vi "OBD_init.vi"(8 "error in":errorcluster, 10 "COM port":refnum<visa-resource-name>="COM2", 11 "cluster input":T1) -> (0 "error out":errorcluster, 2 "OBD enabled":bool=TRUE, 3 "cluster output":T1)   [LabVIEW 2020]
doc: "Initialize OBD communication"
uses:
  controls/StateMachineVariables.ctl
  <vilib>/vision/Avi.llb/IMAQ AVI2 Refnum.ctl
  <vilib>/userDefined/High Color/IMAQdx.ctl
  <vilib>/vision/Deep Learning.llb/IMAQ DL Model Refnum.ctl
  <vilib>/vision/Image Controls.llb/IMAQ Image.ctl
  <vilib>/Instr/_visa.llb/VISA Configure Serial Port (Instr).vi
  terminal_test.vi
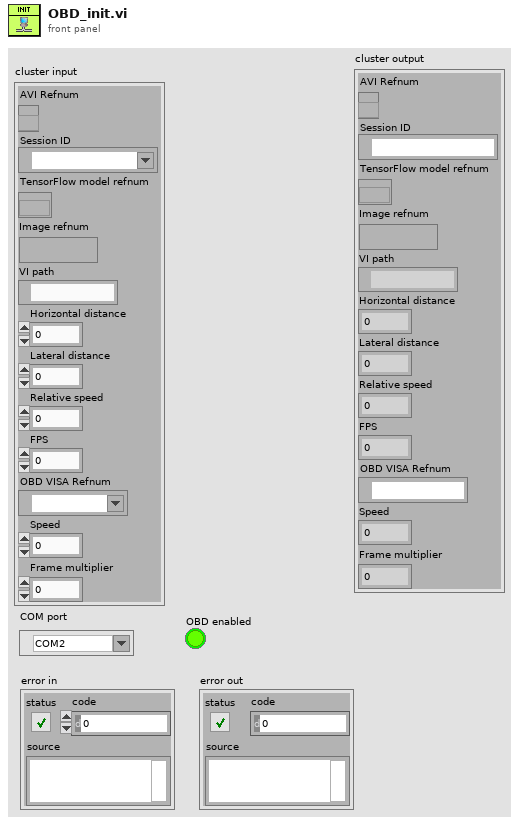
[diagram p1: front panel]
types:
  T1 = typedef "StateMachineVariables.ctl" = cluster{"AVI Refnum":T2, "Session ID":T3, "TensorFlow model refnum":T4, "Image refnum":T5, "VI path":path, "Horizontal distance":dbl, "Lateral distance":dbl, "Relative speed":dbl, "FPS":dbl, "OBD VISA Refnum":refnum<visa-resource-name>, "Speed":dbl, "Frame multiplier":u32}
  T2 = typedef "IMAQ AVI2 Refnum.ctl" = refnum<k20>
  T3 = typedef "IMAQdx.ctl" = refnum<k21>
  T4 = typedef "IMAQ DL Model Refnum.ctl" = refnum<k20>
  T5 = typedef "IMAQ Image.ctl" = refnum<image>
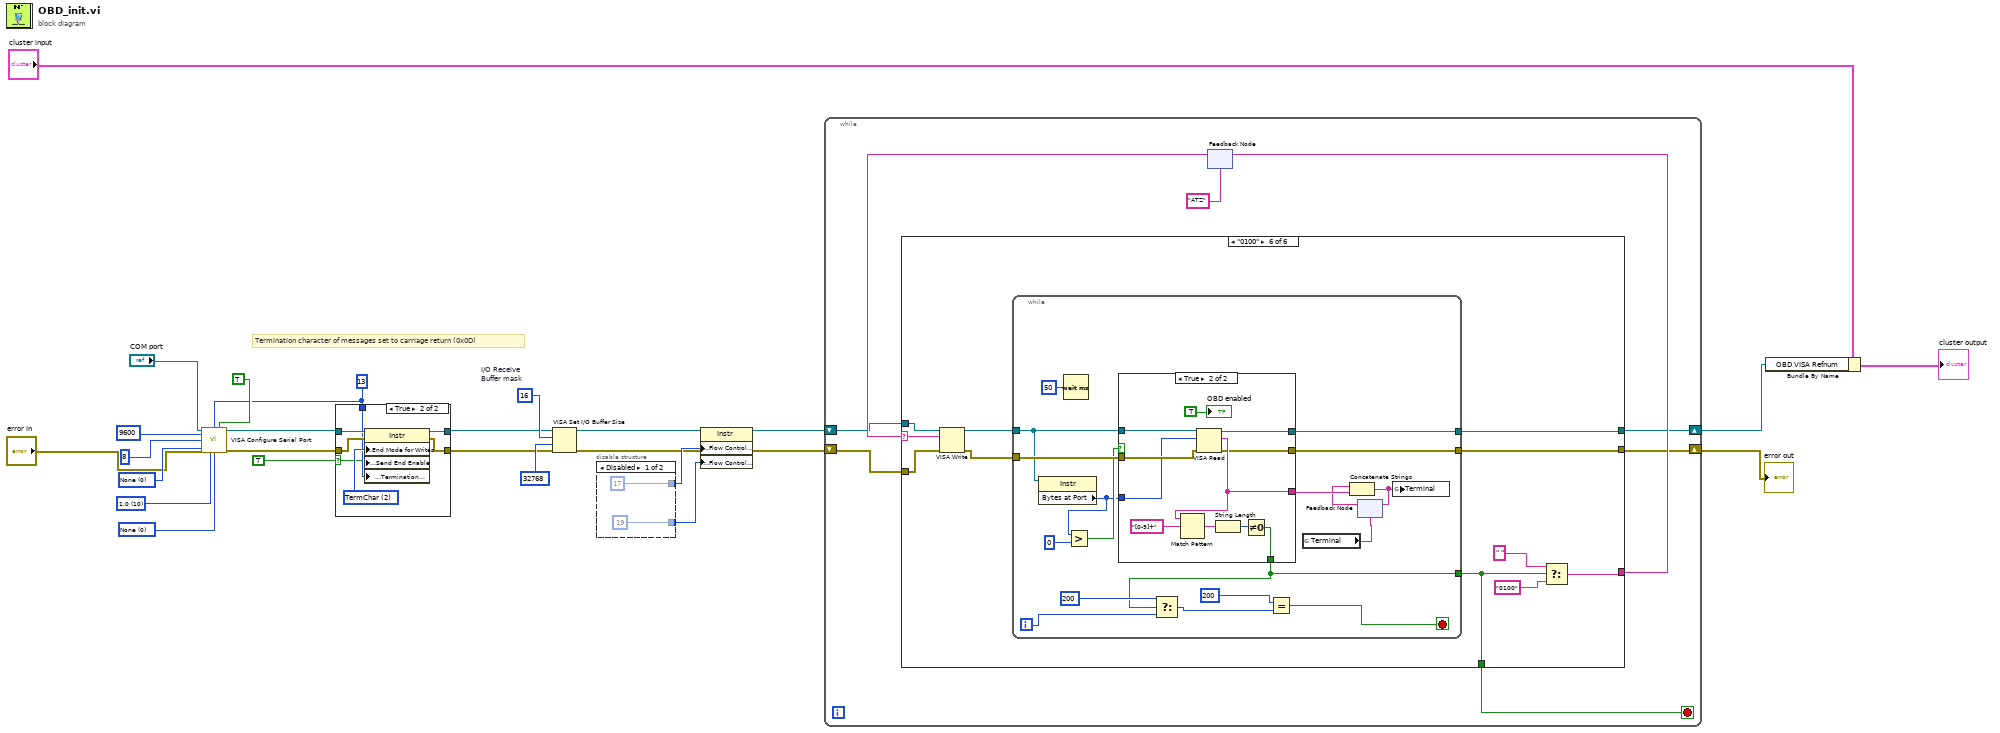
[diagram p0: block diagram]
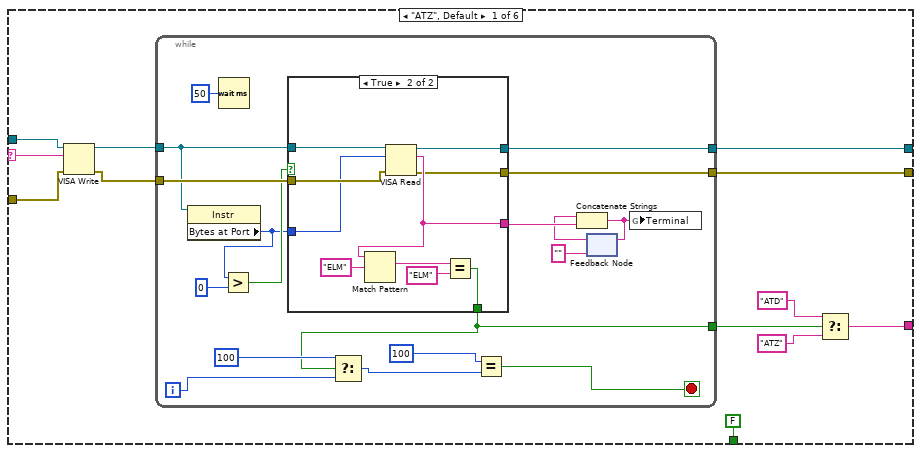
[diagram p4: hidden frame]
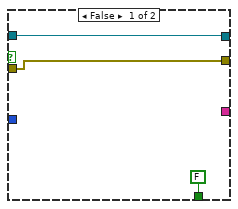
[diagram p5: hidden frame]
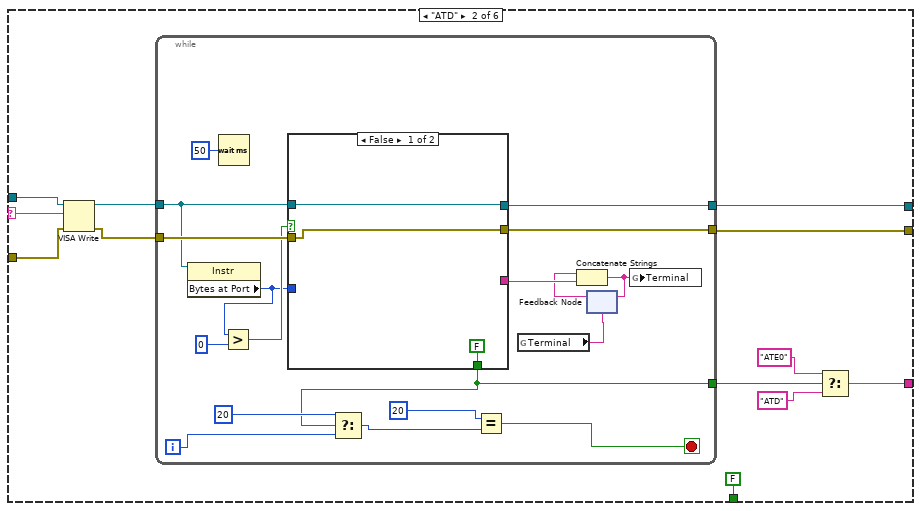
[diagram p6: hidden frame]
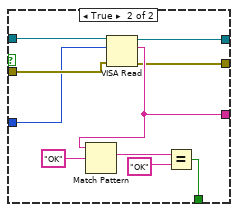
[diagram p7: hidden frame]
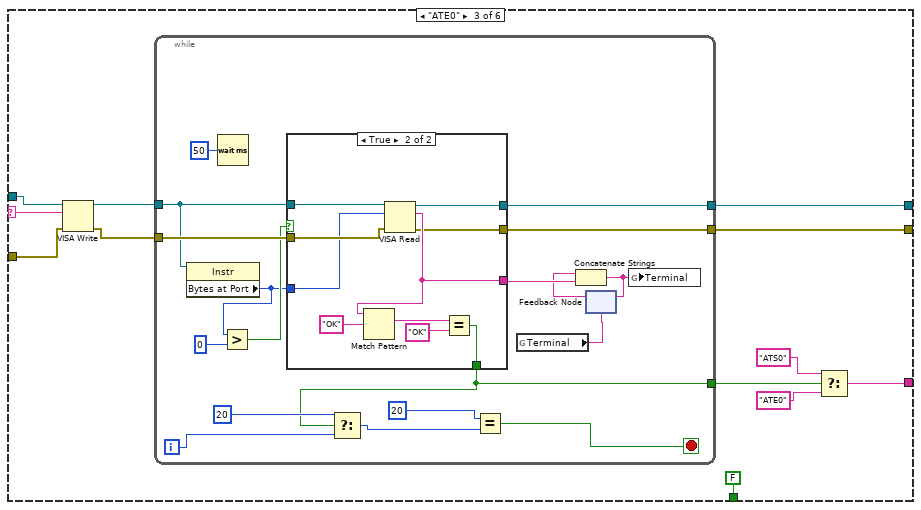
[diagram p8: hidden frame]
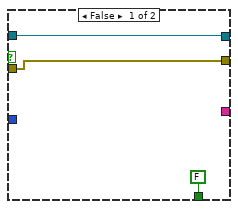
[diagram p9: hidden frame]
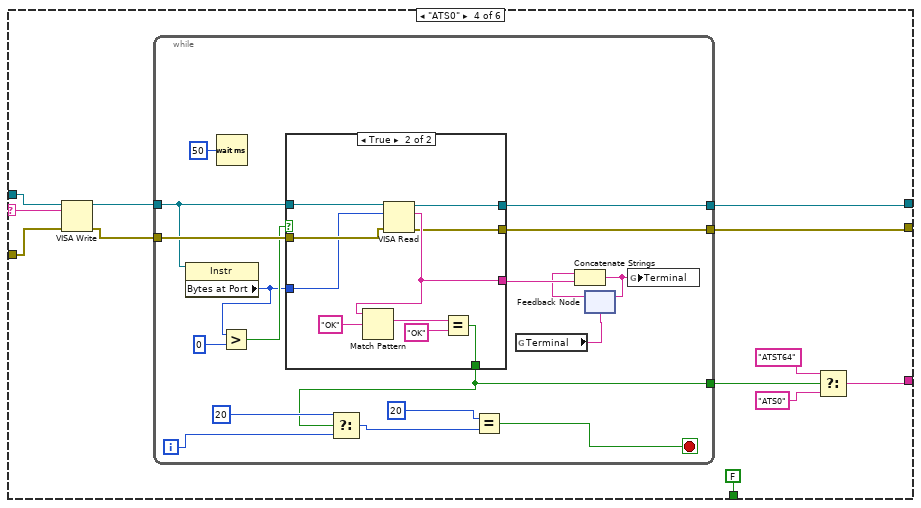
[diagram p10: hidden frame]
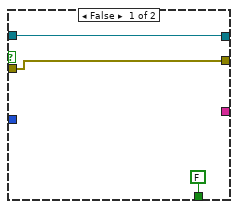
[diagram p11: hidden frame]
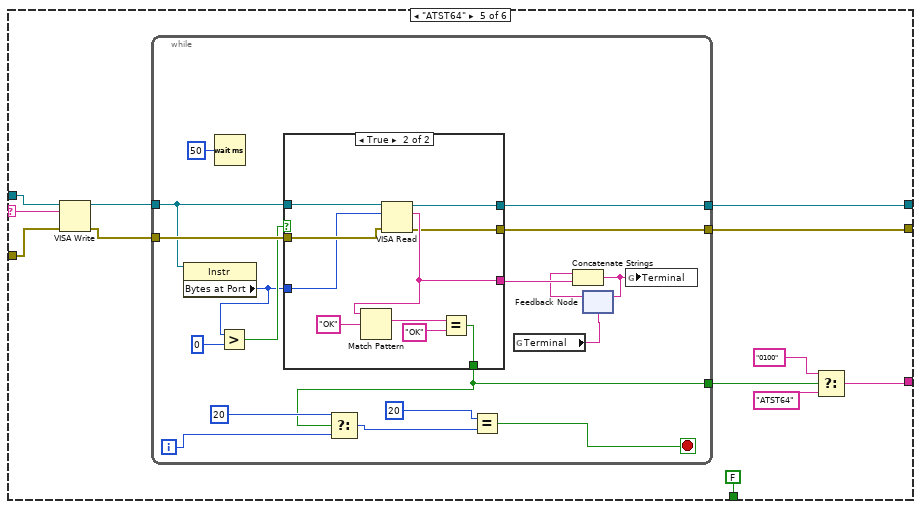
[diagram p12: hidden frame]
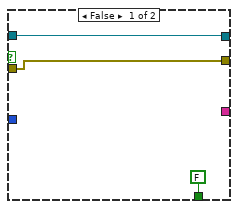
[diagram p13: hidden frame]
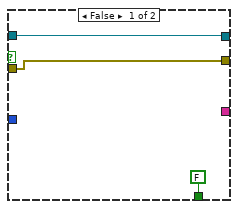
[diagram p14: hidden frame]
diagram:
  w18 = u16 0 items=["None"=0, "XON/XOFF"=1, "RTS/CTS"=2, "DTR/DSR"=4] ("flow control")
  w22 = u16 10 items=["1.0"=10, "1.5"=15, "2.0"=20] ("stop bits")
  w12 = u8 13 ("termination char\n(0xA = '\\n' = LF)")
  w23 = u16 0 items=["None", "Odd", "Even", "Mark", "Space"] ("parity")
  w13 = u16 16  # I/O Receive Buffer mask
  # "Termination character of messages set to carriage return (0x0D)"
  n1 = call-poly "VISA Configure Serial Port"("VISA resource name"="COM port", "termination char\n(0xA = '\\n' = LF)"=w12, "Enable Termination\nChar (T)"=TRUE ("End read on termination character?"), "baud rate (9600)"=u32 9600 ("baud rate"), "data bits (8)"=u16 8 ("data bits"), "parity (0:none)"=w23, "error in (no error)"="error in", "stop bits (10: 1 bit)"=w22, "flow control (0:none)"=w18) -> ("VISA resource name out"=w14:refnum<visa-resource-name>, "error out"=w16:errorcluster)  [unwired: 1 in, 4 out]
  n2 = case shown="True" TRUE ("End write with termination character?") {
    selector: TRUE ("End write with termination character?") -> [_ w28]
    tunnel: w14 -> [w26 w34]
    tunnel: w16 -> [w27 w33]
    tunnel: [w26 w32] -> w8
    tunnel: [w27 w31] -> w15
    tunnel: w12 -> [_ w29]
    frame False {
    }
    frame True {
      w30 = u16 2 items=["None", "LastBit", "TermChar", "Break"] ("Serial Settings:Serial End Mode for Writes")
      n3 = property class="Instr"(reference=w34, error in=w33, "Serial Settings:End Mode for Writes"=w30, "Message Based Settings:Send End Enable"=w28, "Message Based Settings:Termination Character"=w29) -> (reference out=w32:refnum<visa-resource-name>, error out=w31:errorcluster)
    }
  }
  n4 = VISA Set I/O Buffer Size(VISA resource name=w8, mask (16)=w13, size (4096)=u32 32768 ("Input\nbuffer size"), error in (no error)=w15) -> (VISA resource name out=w9:refnum<visa-resource-name>, error out=w6:errorcluster)
  n5 = disable-structure shown="Disabled" {
    disable-tunnel: [u8 17 ("XON Character") _] -> w11
    disable-tunnel: [u8 19 ("XOFF Character") _] -> w10
    frame Disabled {
    }
    frame Enabled {
    }
  }
  n6 = property class="Instr"(reference=w9, "Serial Settings:Flow Control XON Character"=w11, "Serial Settings:Flow Control XOFF Character"=w10) -> (reference out=w5:refnum<visa-resource-name>)  [unwired: 1 in, 1 out]
  n7 = while {
    shift-right: [w39] -> w1
    shift-left: w5 -> [w41]
    shift-right: [w38] -> w25
    shift-left: w6 -> [w40]
    stop <- w37 stop-if-true
    n8 = feedback #1("ATZ") -> (w43:string)
    n9 = case shown="\"0100\"" w43 {
      selector: w43 -> [w56 w92 w134 w178 w218 w265]
      tunnel: [w50 w91 w135 w175 w223 w266] -> w42
      tunnel: w41 -> [w49 w94 w133 w180 w220 w264]
      tunnel: w40 -> [w48 w93 w132 w179 w219 w263]
      tunnel: [w47 w90 w137 w177 w221 w262] -> w39
      tunnel: [w46 w89 w136 w176 w222 w261] -> w38
      tunnel: [FALSE FALSE FALSE FALSE FALSE w260] -> w37
      frame "ATZ", Default {
        n10 = VISA Write(VISA resource name=w49, write buffer=w56, error in (no error)=w48) -> (VISA resource name out=w55:refnum<visa-resource-name>, error out=w54:errorcluster)  [unwired: 1 out]
        n11 = while {
          tunnel: w55 -> [w70]
          tunnel: w54 -> [w74]
          tunnel: [w63] -> w53
          tunnel: [w59] -> w47
          tunnel: [w58] -> w46
          i -> [w67]
          stop <- w66 stop-if-true
          n12 = property class="Instr"(reference=w70) -> ("Bytes at Port"=w71:u32)  [unwired: 1 in, 2 out]
          n13 = Wait (ms)(milliseconds to wait=u32 50) -> ()  [unwired: 1 out]
          n14 = Greater?(x=w71, y=u32 0) -> (0:w72:bool)
          n15 = case shown="True" w72 {
            tunnel: w70 -> [w76 w87]
            tunnel: w74 -> [w75 w86]
            tunnel: w71 -> [_ w85]
            tunnel: [FALSE w81] -> w63
            tunnel: [_ w80] -> w61
            tunnel: [w76 w79] -> w59
            tunnel: [w75 w78] -> w58
            frame False {
            }
            frame True {
              n16 = VISA Read(VISA resource name=w87, byte count=w85, error in (no error)=w86) -> (VISA resource name out=w79:refnum<visa-resource-name>, read buffer=w80:string, error out=w78:errorcluster)  [unwired: 1 out]
              n17 = Match Pattern(string=w80, regular expression="ELM") -> (match substring=w82:string)  [unwired: 1 in, 3 out]
              n18 = Equal?(x=w82, y="ELM") -> (x = y?=w81:bool)
            }
          }
          n19 = Select(t=100, s=w63, f=w67) -> (s? t:f=w65:i32)
          n20 = Equal?(x=100, y=w65) -> (x = y?=w66:bool)
          n21 = feedback #2("") -> (w60:string)
          n22 = Concatenate Strings(w60, w61) -> (w57:string)
          n23 = feedback-in #2(w57) -> ()
          n24 = global write "terminal_test.vi" "Terminal"(w57) -> ()
        }
        n25 = Select(t="ATD", s=w53, f="ATZ") -> (s? t:f=w50:string)
      }
      frame "ATD" {
        n26 = VISA Write(VISA resource name=w94, write buffer=w92, error in (no error)=w93) -> (VISA resource name out=w97:refnum<visa-resource-name>, error out=w98:errorcluster)  [unwired: 1 out]
        n27 = while {
          tunnel: w97 -> [w113]
          tunnel: w98 -> [w117]
          tunnel: [w106] -> w99
          tunnel: [w102] -> w90
          tunnel: [w101] -> w89
          i -> [w110]
          stop <- w109 stop-if-true
          n28 = property class="Instr"(reference=w113) -> ("Bytes at Port"=w114:u32)  [unwired: 1 in, 2 out]
          n29 = Wait (ms)(milliseconds to wait=u32 50) -> ()  [unwired: 1 out]
          n30 = Greater?(x=w114, y=u32 0) -> (0:w115:bool)
          n31 = case shown="False" w115 {
            tunnel: w113 -> [w119 w130]
            tunnel: w117 -> [w118 w129]
            tunnel: w114 -> [_ w128]
            tunnel: [FALSE w124] -> w106
            tunnel: [_ w123] -> w105
            tunnel: [w119 w122] -> w102
            tunnel: [w118 w121] -> w101
            frame False {
            }
            frame True {
              n32 = VISA Read(VISA resource name=w130, byte count=w128, error in (no error)=w129) -> (VISA resource name out=w122:refnum<visa-resource-name>, read buffer=w123:string, error out=w121:errorcluster)  [unwired: 1 out]
              n33 = Match Pattern(string=w123, regular expression="OK") -> (match substring=w125:string)  [unwired: 1 in, 3 out]
              n34 = Equal?(x=w125, y="OK") -> (x = y?=w124:bool)
            }
          }
          n35 = Select(t=20, s=w106, f=w110) -> (s? t:f=w108:i32)
          n36 = Equal?(x=20, y=w108) -> (x = y?=w109:bool)
          n37 = global read "terminal_test.vi" "Terminal"() -> (w100:string)
          n38 = feedback #3(w100) -> (w104:string)
          n39 = Concatenate Strings(w104, w105) -> (w103:string)
          n40 = feedback-in #3(w103) -> ()
          n41 = global write "terminal_test.vi" "Terminal"(w103) -> ()
        }
        n42 = Select(t="ATE0", s=w99, f="ATD") -> (s? t:f=w91:string)
      }
      frame "ATE0" {
        n43 = VISA Write(VISA resource name=w133, write buffer=w134, error in (no error)=w132) -> (VISA resource name out=w142:refnum<visa-resource-name>, error out=w141:errorcluster)  [unwired: 1 out]
        n44 = while {
          tunnel: w142 -> [w156]
          tunnel: w141 -> [w160]
          tunnel: [w149] -> w140
          tunnel: [w145] -> w137
          tunnel: [w144] -> w136
          i -> [w153]
          stop <- w152 stop-if-true
          n45 = property class="Instr"(reference=w156) -> ("Bytes at Port"=w157:u32)  [unwired: 1 in, 2 out]
          n46 = Wait (ms)(milliseconds to wait=u32 50) -> ()  [unwired: 1 out]
          n47 = Greater?(x=w157, y=u32 0) -> (0:w158:bool)
          n48 = case shown="True" w158 {
            tunnel: w156 -> [w162 w173]
            tunnel: w160 -> [w161 w172]
            tunnel: w157 -> [_ w171]
            tunnel: [FALSE w167] -> w149
            tunnel: [_ w166] -> w148
            tunnel: [w162 w165] -> w145
            tunnel: [w161 w164] -> w144
            frame False {
            }
            frame True {
              n49 = VISA Read(VISA resource name=w173, byte count=w171, error in (no error)=w172) -> (VISA resource name out=w165:refnum<visa-resource-name>, read buffer=w166:string, error out=w164:errorcluster)  [unwired: 1 out]
              n50 = Match Pattern(string=w166, regular expression="OK") -> (match substring=w168:string)  [unwired: 1 in, 3 out]
              n51 = Equal?(x=w168, y="OK") -> (x = y?=w167:bool)
            }
          }
          n52 = Select(t=20, s=w149, f=w153) -> (s? t:f=w151:i32)
          n53 = Equal?(x=20, y=w151) -> (x = y?=w152:bool)
          n54 = global read "terminal_test.vi" "Terminal"() -> (w143:string)
          n55 = feedback #4(w143) -> (w147:string)
          n56 = Concatenate Strings(w147, w148) -> (w146:string)
          n57 = feedback-in #4(w146) -> ()
          n58 = global write "terminal_test.vi" "Terminal"(w146) -> ()
        }
        n59 = Select(t="ATS0", s=w140, f="ATE0") -> (s? t:f=w135:string)
      }
      frame "ATS0" {
        n60 = VISA Write(VISA resource name=w180, write buffer=w178, error in (no error)=w179) -> (VISA resource name out=w183:refnum<visa-resource-name>, error out=w184:errorcluster)  [unwired: 1 out]
        n61 = while {
          tunnel: w183 -> [w199]
          tunnel: w184 -> [w203]
          tunnel: [w192] -> w185
          tunnel: [w188] -> w177
          tunnel: [w187] -> w176
          i -> [w196]
          stop <- w195 stop-if-true
          n62 = property class="Instr"(reference=w199) -> ("Bytes at Port"=w200:u32)  [unwired: 1 in, 2 out]
          n63 = Wait (ms)(milliseconds to wait=u32 50) -> ()  [unwired: 1 out]
          n64 = Greater?(x=w200, y=u32 0) -> (0:w201:bool)
          n65 = case shown="True" w201 {
            tunnel: w199 -> [w205 w216]
            tunnel: w203 -> [w204 w215]
            tunnel: w200 -> [_ w214]
            tunnel: [FALSE w210] -> w192
            tunnel: [_ w209] -> w191
            tunnel: [w205 w208] -> w188
            tunnel: [w204 w207] -> w187
            frame False {
            }
            frame True {
              n66 = VISA Read(VISA resource name=w216, byte count=w214, error in (no error)=w215) -> (VISA resource name out=w208:refnum<visa-resource-name>, read buffer=w209:string, error out=w207:errorcluster)  [unwired: 1 out]
              n67 = Match Pattern(string=w209, regular expression="OK") -> (match substring=w211:string)  [unwired: 1 in, 3 out]
              n68 = Equal?(x=w211, y="OK") -> (x = y?=w210:bool)
            }
          }
          n69 = Select(t=20, s=w192, f=w196) -> (s? t:f=w194:i32)
          n70 = Equal?(x=20, y=w194) -> (x = y?=w195:bool)
          n71 = global read "terminal_test.vi" "Terminal"() -> (w186:string)
          n72 = feedback #5(w186) -> (w190:string)
          n73 = Concatenate Strings(w190, w191) -> (w189:string)
          n74 = feedback-in #5(w189) -> ()
          n75 = global write "terminal_test.vi" "Terminal"(w189) -> ()
        }
        n76 = Select(t="ATST64", s=w185, f="ATS0") -> (s? t:f=w175:string)
      }
      frame "ATST64" {
        n77 = VISA Write(VISA resource name=w220, write buffer=w218, error in (no error)=w219) -> (VISA resource name out=w228:refnum<visa-resource-name>, error out=w227:errorcluster)  [unwired: 1 out]
        n78 = while {
          tunnel: w228 -> [w242]
          tunnel: w227 -> [w246]
          tunnel: [w235] -> w226
          tunnel: [w231] -> w221
          tunnel: [w230] -> w222
          i -> [w239]
          stop <- w238 stop-if-true
          n79 = property class="Instr"(reference=w242) -> ("Bytes at Port"=w243:u32)  [unwired: 1 in, 2 out]
          n80 = Wait (ms)(milliseconds to wait=u32 50) -> ()  [unwired: 1 out]
          n81 = Greater?(x=w243, y=u32 0) -> (0:w244:bool)
          n82 = case shown="True" w244 {
            tunnel: w242 -> [w248 w259]
            tunnel: w246 -> [w247 w258]
            tunnel: w243 -> [_ w257]
            tunnel: [FALSE w253] -> w235
            tunnel: [_ w252] -> w234
            tunnel: [w248 w251] -> w231
            tunnel: [w247 w250] -> w230
            frame False {
            }
            frame True {
              n83 = VISA Read(VISA resource name=w259, byte count=w257, error in (no error)=w258) -> (VISA resource name out=w251:refnum<visa-resource-name>, read buffer=w252:string, error out=w250:errorcluster)  [unwired: 1 out]
              n84 = Match Pattern(string=w252, regular expression="OK") -> (match substring=w254:string)  [unwired: 1 in, 3 out]
              n85 = Equal?(x=w254, y="OK") -> (x = y?=w253:bool)
            }
          }
          n86 = Select(t=20, s=w235, f=w239) -> (s? t:f=w237:i32)
          n87 = Equal?(x=20, y=w237) -> (x = y?=w238:bool)
          n88 = global read "terminal_test.vi" "Terminal"() -> (w229:string)
          n89 = feedback #6(w229) -> (w233:string)
          n90 = Concatenate Strings(w233, w234) -> (w232:string)
          n91 = feedback-in #6(w232) -> ()
          n92 = global write "terminal_test.vi" "Terminal"(w232) -> ()
        }
        n93 = Select(t="0100", s=w226, f="ATST64") -> (s? t:f=w223:string)
      }
      frame "0100" {
        n94 = VISA Write(VISA resource name=w264, write buffer=w265, error in (no error)=w263) -> (VISA resource name out=w269:refnum<visa-resource-name>, error out=w270:errorcluster)  [unwired: 1 out]
        n95 = while {
          tunnel: w269 -> [w284]
          tunnel: w270 -> [w288]
          tunnel: [w277] -> w260
          tunnel: [w273] -> w262
          tunnel: [w272] -> w261
          i -> [w281]
          stop <- w280 stop-if-true
          n96 = property class="Instr"(reference=w284) -> ("Bytes at Port"=w285:u32)  [unwired: 1 in, 2 out]
          n97 = Wait (ms)(milliseconds to wait=u32 50) -> ()  [unwired: 1 out]
          n98 = Greater?(x=w285, y=u32 0) -> (0:w286:bool)
          n99 = case shown="True" w286 {
            tunnel: w284 -> [w290 w302]
            tunnel: w288 -> [w289 w301]
            tunnel: w285 -> [_ w300]
            tunnel: [FALSE w299] -> w277
            tunnel: [_ w298] -> w276
            tunnel: [w290 w297] -> w273
            tunnel: [w289 w296] -> w272
            frame False {
            }
            frame True {
              n100 = VISA Read(VISA resource name=w302, byte count=w300, error in (no error)=w301) -> (VISA resource name out=w297:refnum<visa-resource-name>, read buffer=w298:string, error out=w296:errorcluster)  [unwired: 1 out]
              n101 = Match Pattern(string=w298, regular expression="[0-9]+") -> (match substring=w293:string)  [unwired: 1 in, 3 out]
              n102 = String Length(string=w293) -> (length=w294:i32)
              n103 = Not Equal To 0?(x=w294) -> (x != 0?=w299:bool)
              "OBD enabled" <- TRUE
            }
          }
          n104 = Select(t=200, s=w277, f=w281) -> (s? t:f=w279:i32)
          n105 = Equal?(x=200, y=w279) -> (x = y?=w280:bool)
          n106 = global read "terminal_test.vi" "Terminal"() -> (w271:string)
          n107 = feedback #7(w271) -> (w275:string)
          n108 = Concatenate Strings(w275, w276) -> (w274:string)
          n109 = feedback-in #7(w274) -> ()
          n110 = global write "terminal_test.vi" "Terminal"(w274) -> ()
        }
        n111 = Select(t=" ", s=w260, f="0100") -> (s? t:f=w266:string)
      }
    }
    n112 = feedback-in #1(w42) -> ()
  }
  "error out" <- w25
  n113 = Bundle By Name(cluster="cluster input", "OBD VISA Refnum"=w1) -> (→"cluster output":T1)
